vi "single move without gyro.vi"(8 "error in (no error)":errorcluster, 9 "RPM":dbl, 10 "Y":dbl, 11 "X":dbl) -> (0 "error out":errorcluster)   [LabVIEW 2019]
uses:
  <vilib>/Platform/TimedLoop/XDataNode/timing_clust.ctl
  <vilib>/Platform/TimedLoop/XDataNode/nitl_modes.ctl
  <vilib>/Platform/TimedLoop/XDataNode/wakeup.ctl
  <vilib>/platform/TimedLoop/XDataNode/XDataNode.xnode
  <vilib>/Platform/TimedLoop/XDataNode/XDNodeRunTimeDep.lvlib
panel:
  out "Waveform Chart":dbl(graph)
  out "out array":dbl[](array[numeric])
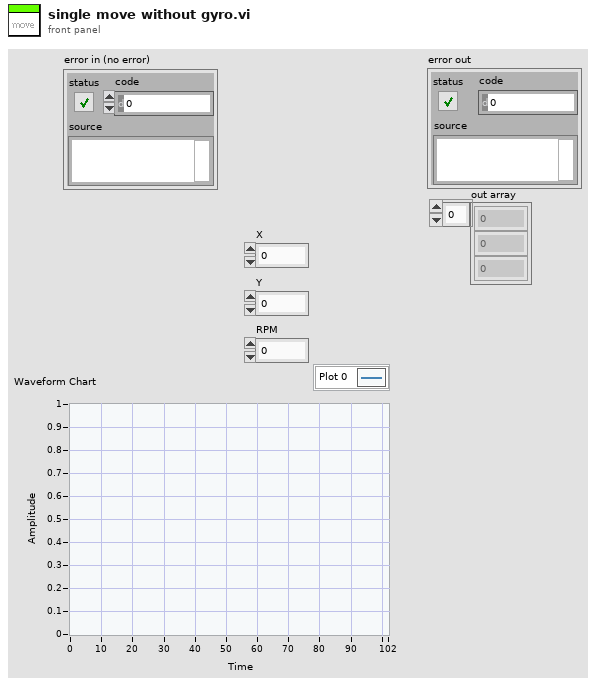
[diagram p1: front panel]
types:
  T1 = typedef "XDNodeRunTimeDep.lvlib/timing_clust.ctl" = cluster{"Expected End [f-1]":u64, "Actual End [f-1]":u64, "Finished Late? [f-1]":bool, "Expected End [i-1]":u64, "Actual End [i-1]":u64, "Finished Late? [i-1]":bool, "Expected Start [i]":u64, "Actual Start [i]":u64, "Expected Start [f]":u64, "Actual Start [f]":u64, "Source Name":string, "Structure Name":string, "Period":i64, "Deadline":i64, "Offset":i64, "Start":i64, "Priority":i32, "Timeout":i32, "Mode":T2, "Wakeup Reason":T3, "Error":errorcluster, "Source Type":string, "Secondary Source Type":string, "Global End Time":u64, "Global Start Time":u64, "Frame Duration":u64, "Iteration Duration":u64, "Assigned CPU":i32, "I/O Scan Engine Mode":u32}
  T2 = typedef "XDNodeRunTimeDep.lvlib/nitl_modes.ctl" = enum32{"No Change", "Process missed periods, maintain original phase", "Discard missed periods, maintain original phase", "Process missed periods, ignore original phase", "Discard missed periods, ignore original phase"}
  T3 = typedef "XDNodeRunTimeDep.lvlib/wakeup.ctl" = enum32{"Normal", "Aborted", "Asynchronous wakeup", "Timing source error", "Timed loop error", "Timeout"}
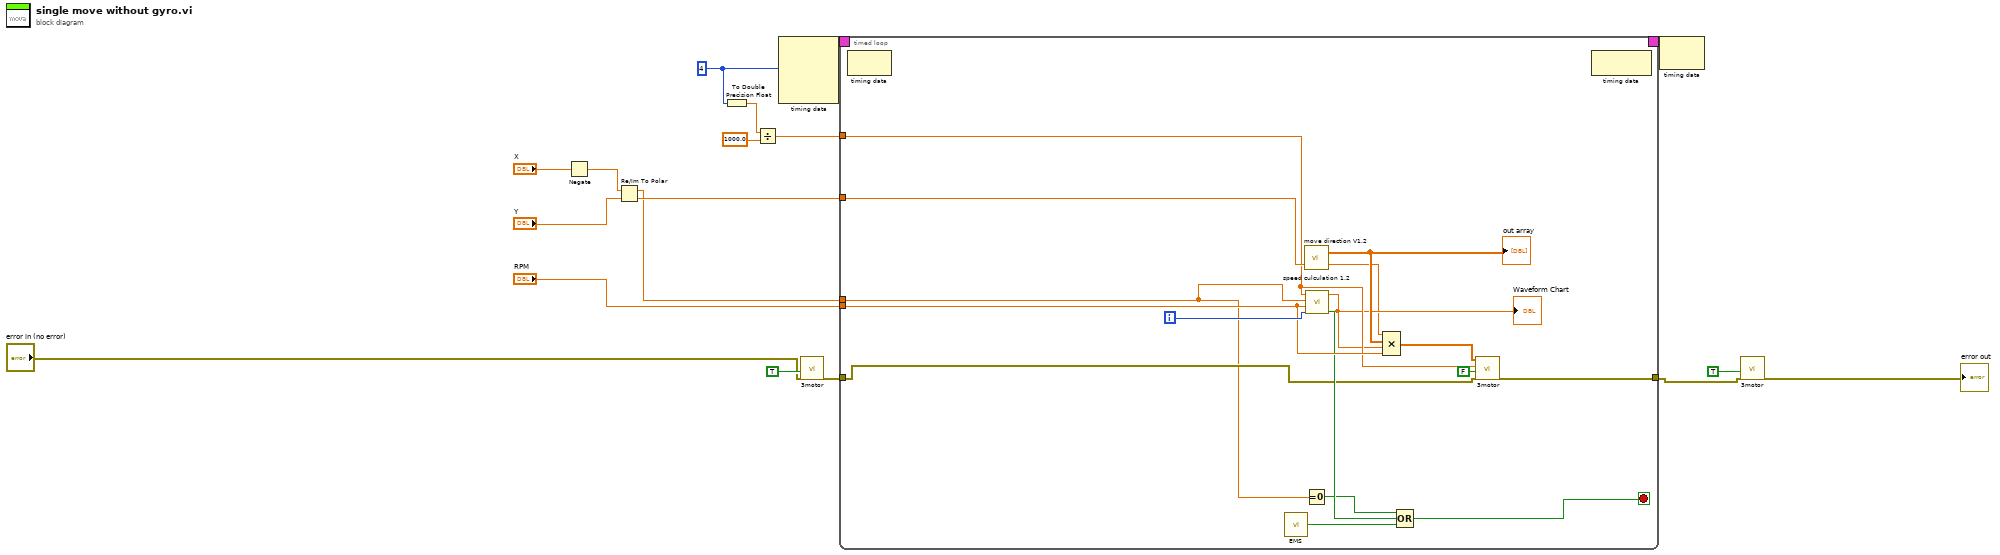
[diagram p0: block diagram]
diagram:
  w16 = i64 4 ("Period")
  n1 = Negate(x="X") -> (-x=w3:dbl)
  n2 = Re/Im To Polar(2:"Y", 3:w3) -> (0:w11:dbl, 1:w10:dbl)
  n3 = To Double Precision Float(number=w16) -> (double precision float=w15:dbl)
  n4 = Divide(x=w15, y=1000.0) -> (x/y=w13:dbl)
  n5 = node-c288(w16) -> (w18:T1)  [unwired: 3 in]
  n6 = call "3motor.vi"("error in (no error)"="error in (no error)", "Reset"=TRUE) -> ("error out"=w8:errorcluster)  [unwired: 8 in, 1 out]
  n7 = timed-loop {
    timing: w18 -> [_]
    timing-out: [_] -> w17
    tunnel: w13 -> [w24]
    tunnel: w11 -> [w33]
    tunnel: w10 -> [w20]
    tunnel: "RPM" -> [w30]
    tunnel: w8 -> [w26]
    tunnel: [w32] -> w2
    i -> [w34]
    stop <- w28 stop-if-true
    n8 = node-c288() -> ()  [unwired: 1 in, 1 out]
    n9 = call "EMS.vi"() -> ("A/DIO4 (Pin 19)"=w25:bool)
    n10 = call "move direction V1.2.vi"("theta"=w33) -> ("max value"=w19:dbl, "out array"=w22:dbl[])  [unwired: 1 in]
    "out array" <- w22
    n11 = Equal To 0?(x=w20) -> (x = 0?=w27:bool)
    n12 = call "speed culculation 1.2.vi"("i"=w34, "Speed(RPM)"=w30, "distance"=w20, "dt(s)"=w24) -> ("complet?"=w29:bool, "Speed"=w21:dbl)  [unwired: 4 in, 2 out]
    "Waveform Chart" <- w21
    n13 = Compound Arithmetic op=MULTIPLY(w19, w22, w21, w30) -> (w31:dbl[])
    n14 = Compound Arithmetic op=OR(w27, w29, w25) -> (w28:bool)
    n15 = call "3motor.vi"("error in (no error)"=w26, "Reset"=FALSE, "dt(s)"=w24, "Motor speed"=w31) -> ("error out"=w32:errorcluster)  [unwired: 6 in, 1 out]
    n16 = node-c288() -> ()  [unwired: 1 in, 1 out]
  }
  n17 = node-c288(w17) -> ()  [unwired: 1 out]
  n18 = call "3motor.vi"("error in (no error)"=w2, "Reset"=TRUE) -> ("error out"=→"error out":errorcluster)  [unwired: 8 in, 1 out]
